vi "New.vi"() -> (0 "error out":errorcluster, 3 "Dummy Motor out":refnum<class "Dummy Motor.lvclass">)   [LabVIEW 2015, in "Dummy Motor.lvclass"]
uses:
  Dummy Motor.lvclass
  Dummy Motor.lvclass/Dummy Motor.ctl
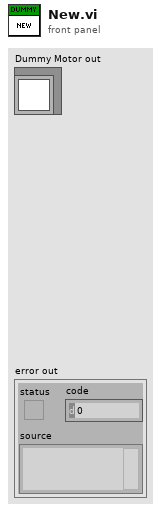
[diagram p1: front panel]
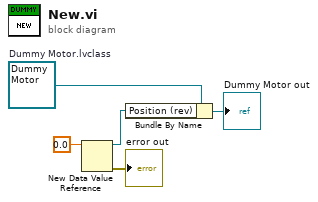
[diagram p0: block diagram]
diagram:
  w4 = refnum<class "Dummy Motor.lvclass"> refnum  # Dummy Motor.lvclass
  n1 = New Data Value Reference(data value=0.0) -> (data value reference=w3:refnum<data-value>, error out=→"error out":errorcluster)  [unwired: 1 in]
  n2 = Bundle By Name(cluster=w4, "Position (rev)"=w3) -> (→"Dummy Motor out":refnum<class "Dummy Motor.lvclass">)
